vi "SS2 Live_Get Ancillary Window Path.vi"(8 "Error In":errorcluster, 11 "SS2 Live Windows":T1) -> (0 "Error Out":errorcluster, 3 "VI Path":path)   [LabVIEW 2019]
uses:
  SS2 Live_Windows List.ctl
  Notebook/Notebook.lvlib
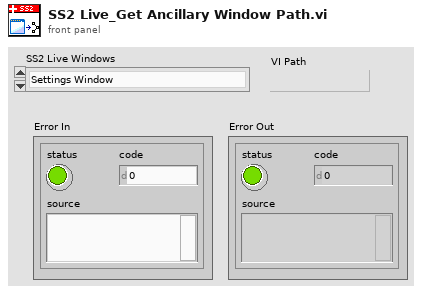
[diagram p1: front panel]
types:
  T1 = typedef "SS2 Live_Windows List.ctl" = enum16{"Settings Window", "Notebook Window", "Histogram Window", "About Window", "SS2 Live Window"}
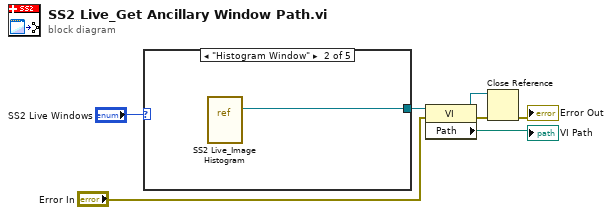
[diagram p0: block diagram]
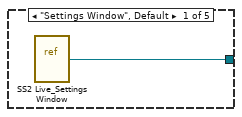
[diagram p2: hidden frame]
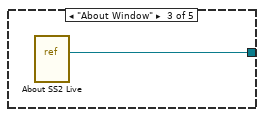
[diagram p3: hidden frame]
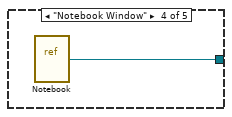
[diagram p4: hidden frame]
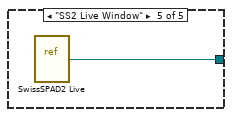
[diagram p5: hidden frame]
diagram:
  n1 = case shown="\"Histogram Window\"" "SS2 Live Windows" {
    tunnel: [w8 w9 w10 w11 w12] -> w6
    frame "Settings Window", Default {
      n2 = vi-ref "SS2 Live_Settings Window.vi"() -> (w8:refnum<vi>)
    }
    frame "Histogram Window" {
      n3 = vi-ref "SS2 Live_Image Histogram.vi"() -> (w9:refnum<vi>)
    }
    frame "About Window" {
      n4 = vi-ref "About SS2 Live.vi"() -> (w10:refnum<vi>)
    }
    frame "Notebook Window" {
      n5 = vi-ref "Notebook.vi"() -> (w11:refnum<vi>)
    }
    frame "SS2 Live Window" {
      n6 = vi-ref "SwissSPAD2 Live.vi"() -> (w12:refnum<vi>)
    }
  }
  n7 = property class="VI"(reference=w6, error in="Error In") -> (reference out=w4:refnum<vi>, error out=w5:errorcluster, "Path"=→"VI Path":path)
  n8 = Close Reference(reference=w4, error in (no error)=w5) -> (error out=→"Error Out":errorcluster)
